vi "Actor Core.vi"(8 "error in":errorcluster, 11 "Channel Selector in":refnum<class "VF Device Selection.lvclass">) -> (0 "error out":errorcluster, 3 "Actor out":refnum<class "Actor.lvclass">)   [LabVIEW 2018, in "VF Device Selection Actor.lvlib" / "VF Device Selection.lvclass"]
doc: "(<B>Filename</B>: Actor Framework.lvlib:Actor.lvclass:Actor Core.vi)\n\nReceives messages to the actor, reacts to them, and initiates any error handling that may shut the actor down.\n\nDescendant classes may override this VI to append parallel tasks for the actor to complete while it handles messages. Overrides use the Call Parent Method node."
uses:
  VF Device Selection.lvclass
  C:/Program Files (x86)/National Instruments/LabVIEW 2018/vi.lib/ActorFramework/Actor/Actor.lvclass
  <vilib>/ActorFramework/Actor/Actor.lvclass
  VF Device Selection.lvclass/VF Device Selection.ctl
  <vilib>/ActorFramework/Actor/Actor.lvclass/Actor.ctl
  <vilib>/ActorFramework/Message Enqueuer/Message Enqueuer.lvclass/Message Enqueuer.ctl
  EMS User Interface Actor/EMS User Interface Messages/Write VF Device ID Msg/Write VF Device ID Msg.lvclass/Write VF Device ID Msg.ctl
  <vilib>/ActorFramework/Message Enqueuer/Init from Existing Queue.vi
  <vilib>/ActorFramework/Message Enqueuer/Enqueue.vi
  <vilib>/ActorFramework/Stop Msg/Stop Msg.lvclass
  C:/Program Files (x86)/National Instruments/LabVIEW 2018/vi.lib/ActorFramework/Message/Message.lvclass
  EMS User Interface Actor/EMS User Interface Messages/Write VF Device ID Msg/Write VF Device ID Msg.lvclass
  <vilib>/ActorFramework/Message Priority Queue/Priority Enqueue.vi
  <vilib>/ActorFramework/Message Enqueuer/Message Enqueuer.lvclass
panel:
  in  "Cancel Button":bool
  in  "OK Button":bool
  in  "Channels":i32[](listbox)
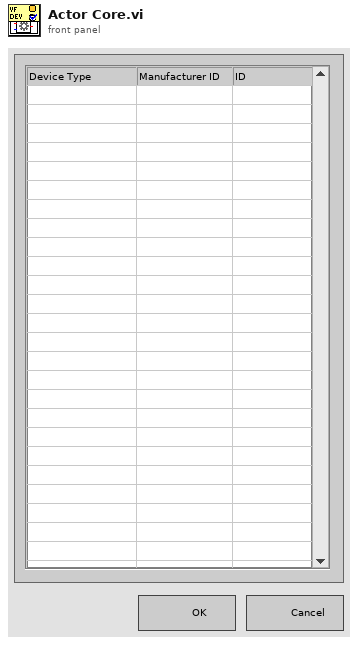
[diagram p1: front panel]
types:
  T1 = enum32{"Invalid", "Standard", "Closed", "Hidden", "Minimized", "Maximized"}
  T2 = typedef "VF Device Selection Actor.lvlib/VF Device Selection.lvclass/VF Device Selection User Events.ctl" = cluster{"ItemNames":refnum<user-event>, "stop":refnum<user-event>}
  T3 = typedef "CSEISMIC DDS.lvlib/CSEISMIC DDS.lvclass/DeviceID.ctl" = string
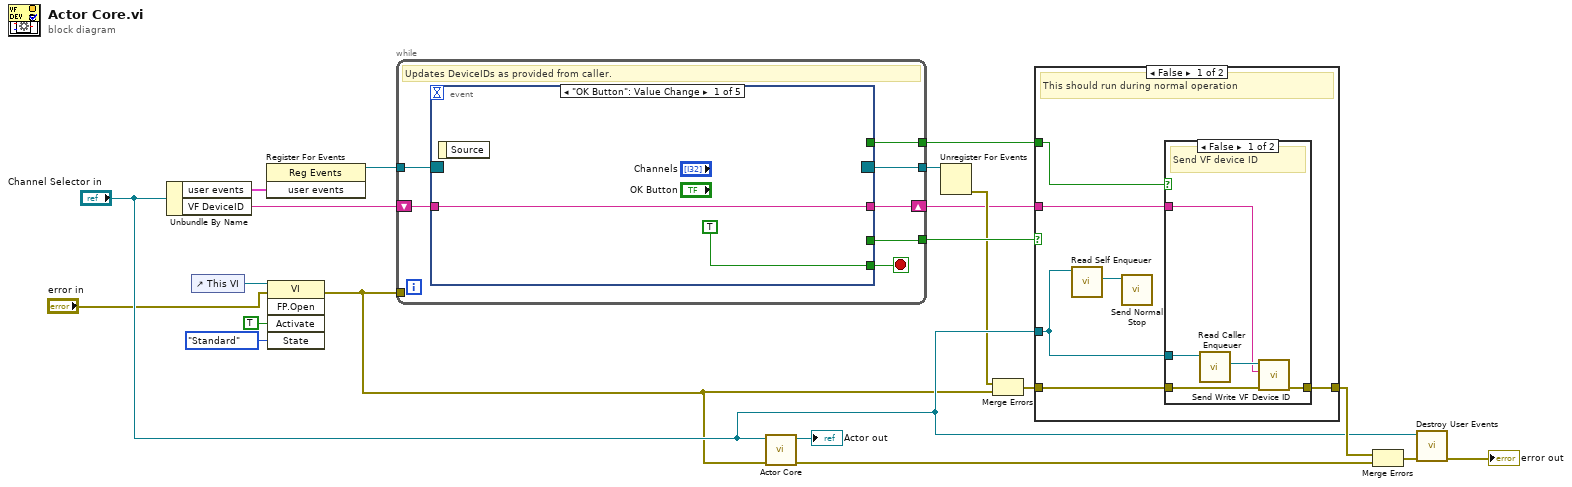
[diagram p0: block diagram]
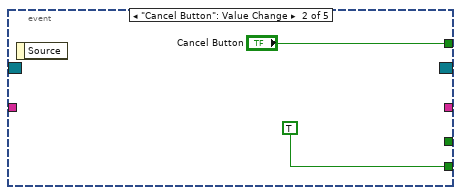
[diagram p4: hidden frame]
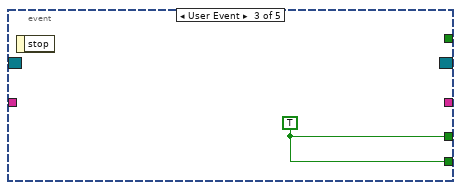
[diagram p5: hidden frame]
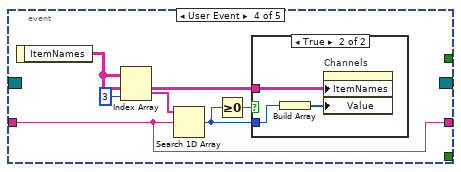
[diagram p6: hidden frame]
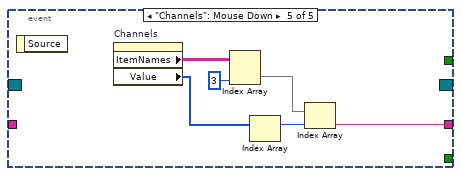
[diagram p8: hidden frame]
diagram:
  n1 = Unbundle By Name("Channel Selector in") -> ("user events"=w17:T2, "VF DeviceID"=w1:T3)
  n2 = control-ref of="This VI"() -> (w8:refnum<vi>)
  n3 = register-events(w17) -> (reference out=w16:refnum<event-registration>)  [unwired: 2 in, 1 out]
  n4 = invoke class="VI" method="FP.Open"(reference=w8, error in="error in", "Activate"=TRUE ("Activate?"), "State"=T1."Standard") -> (error out=w4:errorcluster)  [unwired: 1 in, 4 out]
  n5 = while {
    tunnel: w16 -> [w26]
    tunnel: [w25] -> w15
    tunnel: [w24] -> w12
    tunnel: w4 -> [_]
    shift-right: [w23] -> w2
    shift-left: w1 -> [w22]
    tunnel: [w21] -> w3
    stop <- w27 stop-if-true
    # "Updates DeviceIDs as provided from caller."
    n6 = event shown="[0] \"OK Button\": Value Change" {
      selector: w26 -> [_ _ _ _ _]
      dyn-events: [_ _ _ _ _] -> w25
      timeout: _ -> [_ _ _ _ _]
      tunnel: [TRUE TRUE w32 _ _] -> w27
      tunnel: [_ _ w32 _ _] -> w24
      tunnel: [w28 _ _ w33 w42] -> w23
      tunnel: w22 -> [w28 _ _ w33 _]
      tunnel: [_ "Cancel Button" _ _ _] -> w21
      event "OK Button": Value Change {
        n7 = event-data() -> ()  [unwired: 1 in, 1 out]
      }
      event "Cancel Button": Value Change {
        n8 = event-data() -> ()  [unwired: 1 in, 1 out]
      }
      event User Event {
        w32 = TRUE
        n9 = event-data() -> ()  [unwired: 1 in, 1 out]
      }
      event User Event {
        n10 = event-data() -> ("ItemNames"=w37:string[][])  [unwired: 1 in]
        n11 = Index Array(array=w37, index (col)=3 ("disabled index (col)")) -> (element=w35:string[])  [unwired: 1 in]
        n12 = Search 1D Array(1D array=w35, element=w33) -> (index of element=w36:i32)  [unwired: 1 in]
        n13 = Greater Or Equal To 0?(x=w36) -> (x >= 0?=w34:bool)
        n14 = case shown="True" w34 {
          tunnel: w37 -> [_ w41]
          tunnel: w36 -> [_ w40]
          frame False {
          }
          frame True {
            n15 = Build Array(w40) -> (w39:i32[])
            n16 = property on="Channels" class="MCListbox (strict)"("ItemNames"=w41, "Value"=w39) -> ()  [unwired: 2 in, 2 out]
          }
        }
      }
      event "Channels": Mouse Down {
        n17 = event-data() -> ()  [unwired: 1 in, 1 out]
        n18 = property on="Channels" class="MCListbox (strict)"() -> ("ItemNames"=w46:string[][], "Value"=w45:i32[])  [unwired: 2 in, 2 out]
        n19 = Index Array(array=w46, index (col)=3 ("disabled index (col)")) -> (element=w44:string[])  [unwired: 1 in]
        n20 = Index Array(array=w45) -> (element=w43:i32)  [unwired: 1 in]
        n21 = Index Array(array=w44, index=w43) -> (element=w42:string)
      }
    }
  }
  n22 = call-parent "Actor Core.vi"("error in"=w4, "Actor in"="Channel Selector in") -> ("error out"=w20:errorcluster, "Actor out"=→"Actor out":refnum<class "Actor.lvclass">)  [unwired: 8 in]
  n23 = Unregister For Events(event registration refnum=w15) -> (error out=w9:errorcluster)  [unwired: 1 in]
  n24 = Merge Errors(w9, w4) -> (w10:errorcluster)
  n25 = case shown="False" w12 {
    tunnel: [w50 w60] -> w18
    tunnel: w10 -> [w51 w60]
    tunnel: "Channel Selector in" -> [w52 _]
    tunnel: w3 -> [w48 _]
    tunnel: w2 -> [w49 _]
    frame False {
      # "This should run during normal operation"
      n26 = call <vilib>:"Read Self Enqueuer.vi"("Actor"=w52) -> ("Self Enqueuer"=w53:refnum<class "Message Enqueuer.lvclass">)  [unwired: 10 in]
      n27 = call <vilib>:"Send Normal Stop.vi"("Message Enqueuer"=w53) -> ()  [unwired: 10 in, 1 out]
      n28 = case shown="False" w48 {
        tunnel: w52 -> [w58 _]
        tunnel: w51 -> [w55 w59]
        tunnel: [w54 w59] -> w50
        tunnel: w49 -> [w56 _]
        frame False {
          # "Send VF device ID"
          n29 = call <vilib>:"Read Caller Enqueuer.vi"("Actor"=w58) -> ("Caller Enqueuer"=w57:refnum<class "Message Enqueuer.lvclass">)  [unwired: 10 in]
          n30 = call "Send Write VF Device ID.vi"("error in (no error)"=w55, "VF Device ID"=w56, "Message Enqueuer"=w57) -> ("error out"=w54:errorcluster)  [unwired: 7 in, 1 out]
        }
        frame True {
          # "Cancelled"
        }
      }
    }
    frame True {
      # "This executes when the actor is stopped programmatically rather than through the UI."
    }
  }
  n31 = Merge Errors(w18, w20) -> (w14:errorcluster)
  n32 = call "Destroy User Events.vi"("error in"=w14, "VF Device Selection in"="Channel Selector in") -> ("error out"=→"error out":errorcluster)  [unwired: 8 in, 1 out]
